vi "Check Star Time.vi"(8 "error in (no error)":errorcluster, 11 "Star in":refnum<class "Star.lvclass">) -> (0 "error out":errorcluster, 3 "Star out":refnum<class "Star.lvclass">)   [LabVIEW 2021, in "Star.lvclass"]
uses:
  Star.lvclass
  C:/Users/poche/Programs/LabVIEW/imposible snake/GameEl_class/GameEl.lvclass
  Star.lvclass/Star.ctl
  GameEl_class/GameEl.lvclass/GameEl.ctl
  GameEl_class/GameEl.lvclass
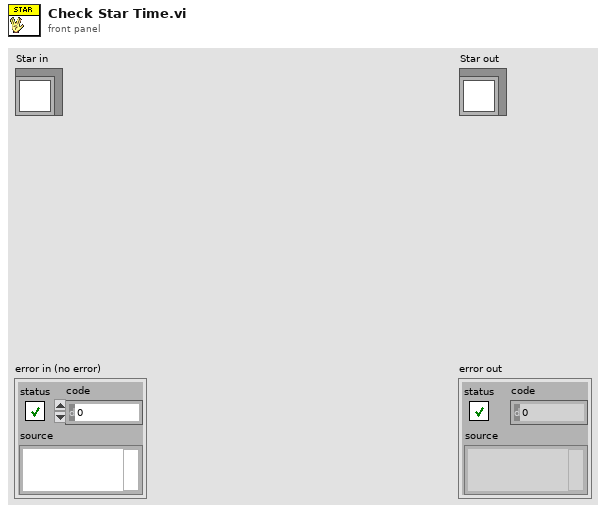
[diagram p1: front panel]
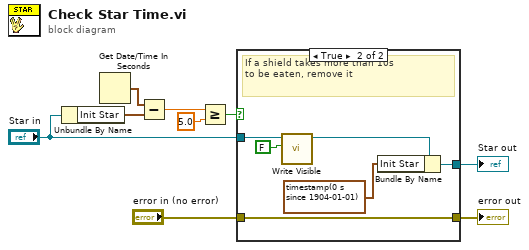
[diagram p0: block diagram]
diagram:
  n1 = Unbundle By Name("Star in") -> ("Init Star"=w6:timestamp)
  n2 = Get Date/Time In Seconds() -> (seconds since 1Jan1904=w7:timestamp)
  n3 = Subtract(x=w7, y=w6) -> (x-y=w5:dbl)
  n4 = Greater Or Equal?(x=w5, y=5.0) -> (x >= y?=w3:bool)
  n5 = case shown="True" w3 {
    tunnel: "Star in" -> [w11 w17]
    tunnel: [w11 w16] -> w8
    tunnel: "error in (no error)" -> [w10 w14]
    tunnel: [w10 w14] -> w1
    frame False {
    }
    frame True {
      # "If a shield takes more than 10s\nto be eaten, remove it"
      n6 = call "Write Visible.vi"("Visible"=FALSE, "GameEl in"=w17) -> ("GameEl out"=w13:refnum<class "Star.lvclass">)  [unwired: 8 in, 1 out]
      n7 = Bundle By Name(cluster=w13, "Init Star"=timestamp(0 s since 1904-01-01) ("Init Shield")) -> (w16:refnum<class "Star.lvclass">)
    }
  }
  "error out" <- w1
  "Star out" <- w8
